vi "Update New Versions.vi"(8 "Error In":errorcluster, 9 "Index Array":i32[][](array[numeric]), 10 "New Version":string[](array[string]), 11 "Tab Page Ref":refnum<vi>[](array[refnum])) -> (0 "Error Out":errorcluster, 2 "New Version dup":string[](array[string]))   [LabVIEW 2014]
doc: "This VI gets the 1D array New Version and 2D array Index Array. It updates the new configuration array on each page of the tab control."
panel:
  out "Array":i32[](array[numeric])
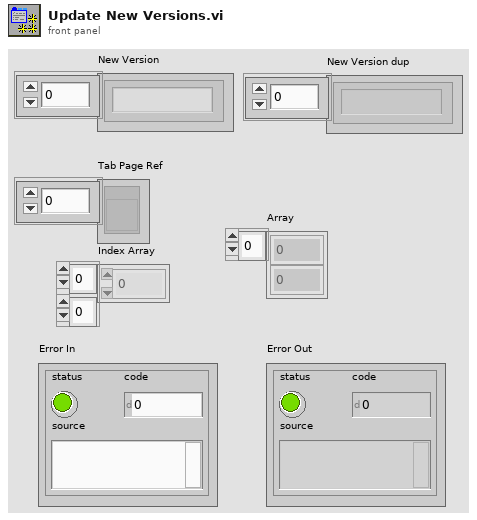
[diagram p1: front panel]
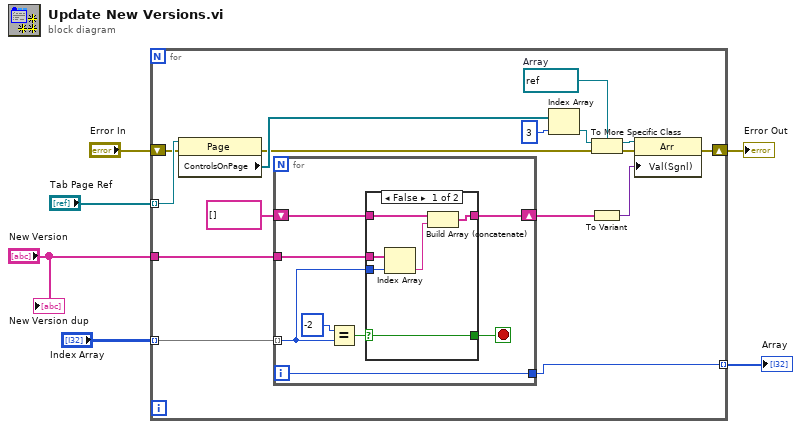
[diagram p0: block diagram]
diagram:
  n1 = for {
    tunnel: "Tab Page Ref" -> [w22] mode=indexing
    shift-right: [w9] -> w4
    shift-left: "Error In" -> [w21]
    tunnel: "New Version" -> [w12]
    tunnel: "Index Array" -> [w13] mode=indexing
    tunnel: [w7] -> w1 mode=indexing
    w14 = refnum<vi> refnum  # Array
    n2 = property class="Page"(reference=w22, error in=w21) -> (error out=w17:errorcluster, "ControlsOnPage"=w20:refnum<vi>[])  [unwired: 1 out]
    n3 = for {
      tunnel: w13 -> [w27] mode=indexing
      tunnel: w12 -> [w30]
      shift-right: [w25] -> w11
      shift-left: string[] [] -> [w26]
      tunnel: [w23] -> w7
      i -> [w23]
      stop <- w24 stop-if-true
      n4 = Equal?(x=-2, y=w27) -> (x = y?=w28:bool)
      n5 = case shown="False" w28 {
        selector: w28 -> [w34 w37]
        tunnel: w30 -> [w36 _]
        tunnel: w27 -> [w35 _]
        tunnel: w26 -> [w33 w38]
        tunnel: [w31 w38] -> w25
        tunnel: [w34 w37] -> w24
        frame False {
          n6 = Index Array(array=w36, index=w35) -> (element=w32:string)
          n7 = Build Array (concatenate)(w33, w32) -> (w31:string[])
        }
        frame True {
        }
      }
    }
    n8 = Index Array(array=w20, index=3) -> (element=w16:refnum<vi>)
    n9 = To More Specific Class(target class=w14, reference=w16, error in=w17) -> (specific class reference=w15:refnum<vi>, error out=w18:errorcluster)
    n10 = To Variant(anything=w11) -> (Variant=w10:variant)
    n11 = property class="Arr"(reference=w15, error in=w18, "Val(Sgnl)"=w10) -> (error out=w9:errorcluster)  [unwired: 1 out]
  }
  "Error Out" <- w4
  "Array" <- w1
  "New Version dup" <- "New Version"
